vi "NI VeriStand - Get Fault Value.vi"(8 "error in (no error)":errorcluster, 10 "Channel":string, 11 "ChannelFault in":T1) -> (0 "error out":errorcluster, 1 "Fault Value":dbl, 2 "Faulted":bool, 3 "ChannelFault out":T1)   [LabVIEW 2020, in "NI_VS ChannelFault ExecutionAPI.lvlib"]
doc: "Returns the fault value of the specified channel."
uses:
  <vilib>/NI VeriStand/Execution/ChannelFaultManager/NI_VS ChannelFault ExecutionAPI.lvlib
  <vilib>/NI VeriStand/Execution/ChannelFaultManager/ChannelFaultAPI.ctl
  NationalInstruments.VeriStand.ClientAPI
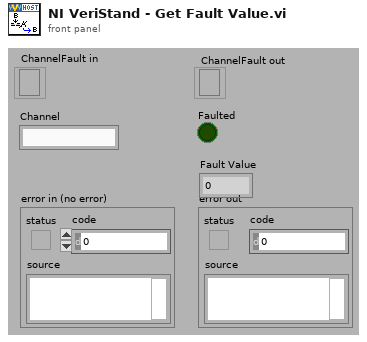
[diagram p1: front panel]
types:
  T1 = typedef "NI_VS ChannelFault ExecutionAPI.lvlib/ChannelFaultAPI.ctl" = refnum<k24>
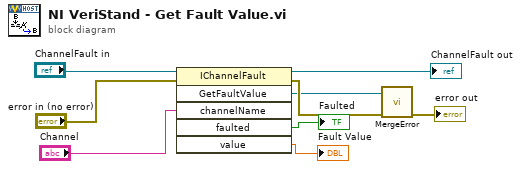
[diagram p0: block diagram]
diagram:
  n1 = invoke class="IChannelFault" method="GetFaultValue"(reference="ChannelFault in", error in="error in (no error)", "channelName"="Channel") -> (reference out=→"ChannelFault out":T1, error out=w7:errorcluster, "GetFaultValue"=w6:refnum<k24>, "faulted"=→"Faulted":bool, "value"=→"Fault Value":dbl)  [unwired: 3 in, 1 out]
  n2 = call <vilib>:"MergeError.vi"("error in (no error)"=w7, "Error"=w6) -> ("error out"=→"error out":errorcluster)  [unwired: 9 out]
